vi "q3 array.vi"() -> ()   [LabVIEW 2018]
panel:
  out "Array 2":dbl[](array[numeric])
  in  "t":dbl
  in  "Array":dbl[](array[numeric])
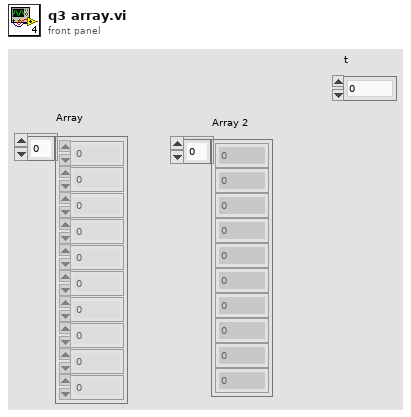
[diagram p1: front panel]
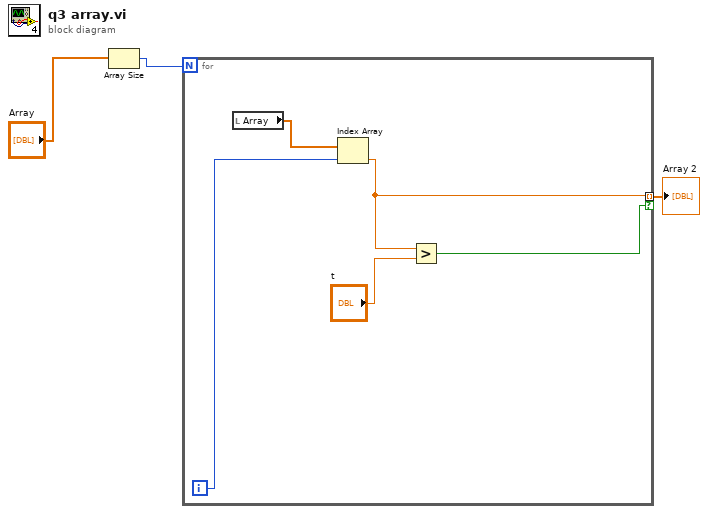
[diagram p0: block diagram]
diagram:
  n1 = Array Size(array="Array") -> (size(s)=w3:i32)
  n2 = for {
    N: w3 -> [_]
    tunnel: [w5] -> w1 mode=indexing if=w4
    i -> [w8]
    n3 = local read "Array"() -> (w7:dbl[])
    n4 = Index Array(array=w7, index=w8) -> (element=w5:dbl)
    n5 = Greater?(x=w5, y="t") -> (0:w4:bool)
  }
  "Array 2" <- w1
